vi "Swerve Drive 2 Controller.vi"(8 "error in":errorcluster) -> ()   [LabVIEW 2015]
doc: "This VI executes continuously carrying out the current operation and responding to updates or new operations. It will often contain the timing or control code that is difficult to place directly in TeleOp. This VI generally opens all sensors and motors and isolates the rest of the robot code from knowing how the operations are carried out."
uses:
  <vilib>/Utility/config.llb/NI_LVConfig.lvlib
  <vilib>/Rock Robotics/WPI/CAN/TalonSRX/WPI_CANTalonSRX_APIFeedbackSelect.ctl
  <vilib>/Rock Robotics/WPI/CAN/TalonSRX/WPI_CANTalonSRX_APIControlMode.ctl
  <vilib>/Rock Robotics/WPI/MotorControl/WPI_MotorControlOpenCANTalonSRX.vi
  navX/navX Library v2/navX Library v2.lvlib
  Swerve Drive 2 Operations.ctl
  Swerve Drive 2 Setpoints.ctl
  <vilib>/Utility/config.llb/Read Key (Double).vi
  navX/navX Library v2/IO/Open/Z900_navX_Open_SPI.vi
  <vilib>/Rock Robotics/Network Tables/NT Write Boolean.vi
panel:
  in  "Absolute Encoder TPR":dbl
  out "Joystick":T1
  in  "Speed PID":cluster{"P":dbl, "I":dbl, "D":dbl}={"P"=48.0, "I"=0.0, "D"=638.0}
  in  "Ramp Rate":dbl=50.0
  in  "Steering PID":cluster{"P":dbl, "I":dbl, "D":dbl}={"P"=0.0275, "I"=0.000115, "D"=0.682955}
  out "Current\nCmd":string
  # "Tip: It may be helpful to observe inputs and sensor values.\nYou may also want to display tuning or debugging controls."
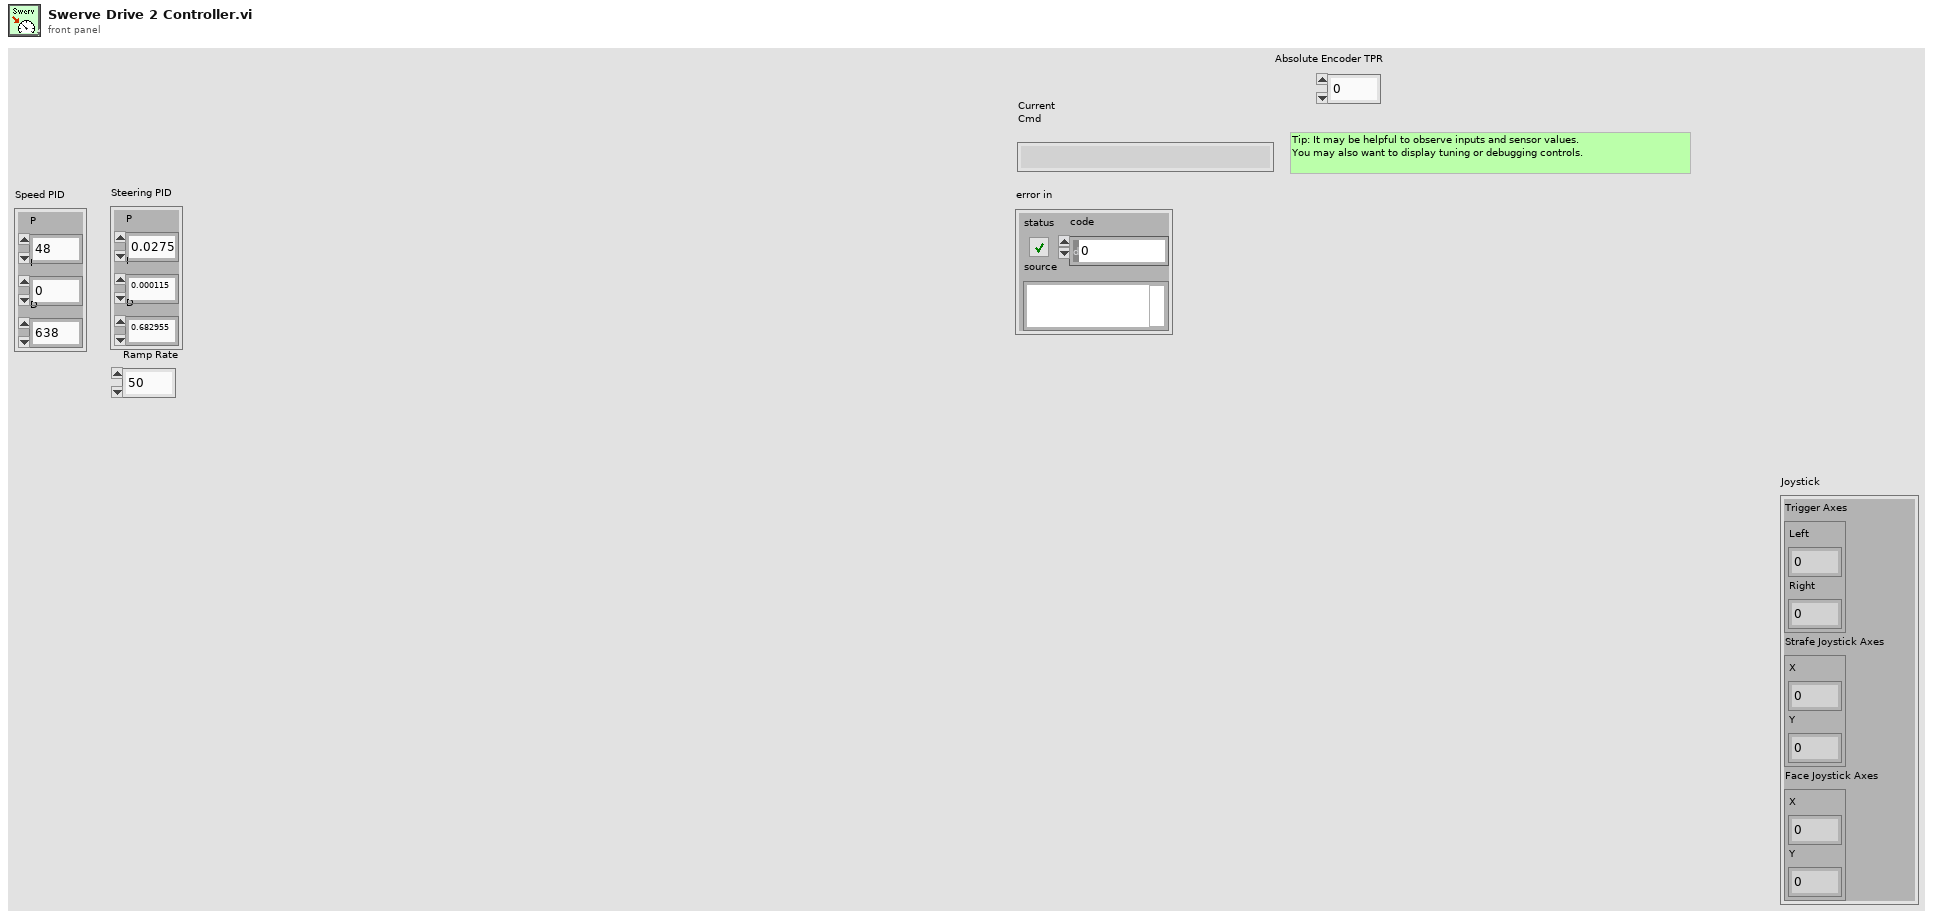
[diagram p1: front panel]
types:
  T1 = cluster{"Trigger Axes":cluster{"Left":dbl, "Right":dbl}, "Strafe Joystick Axes":cluster{"X":dbl, "Y":dbl}, "Face Joystick Axes":cluster{"X":dbl, "Y":dbl}}
  T2 = typedef "Swerve Drive 2 Setpoints.ctl" = cluster{"Operation":T3, "Duration":dbl, "Speed Multiplier":dbl, "Joystick":cluster{"Trigger Axes":cluster{"Left":dbl, "Right":dbl}, "Strafe Joystick Axes":cluster{"X":dbl, "Y":dbl}, "Face Joystick Axes":cluster{"X":dbl, "Y":dbl}}, "Position":cluster{"X":dbl, "Y":dbl, "R":dbl}}
  T3 = typedef "Swerve Drive 2 Operations.ctl" = enum16{"Reserve", "Read Current", "Immeditate", "Drive", "Go to Coordinates"}
  T4 = typedef "NI_LVConfig.lvlib/Config Data RefNum.ctl" = refnum<k1>
  T5 = typedef "WPI_CANTalonSRX_APIFeedbackSelect.ctl" = enum16{"Digital Quadrature Encoder", "Analog Potentiometer", "Analog Encoder", "Count on Quad-A (Rising-Edge)", "Count on Quad-A (Falling-Edge)", "CTR Magnetic Enc (Absolute)", "CTR Magnetic Enc (Relative)", "Pulse Width"}
  T6 = typedef "WPI_CANTalonSRX_APIControlMode.ctl" = enum8{"Percent VBus", "Speed", "Position", "Slave", "Unchanged / Invalid", "Voltage Compensation", "Current"}
  T7 = typedef "WPI_MotorControlDeviceRef.ctl" = cluster{"DeviceStatus":errorcluster, "Type":T8, "PWM":cluster{"PWM Channel":T9, "DeadBand":T10}, "CAN":cluster{"Device Number":u8, "Control Mode":T11, "Semaphore":T12, "Max Vout":dbl, "TalonSRX Control Mode":T6}, "Invert":bool}
  T8 = typedef "WPI_MotorControlType.ctl" = enum16{"PWM", "CAN", "CANTalonSRX"}
  T9 = typedef "FPGA_DIOPWMChannel.ctl" = enum8{"PWM 0", "PWM 1", "PWM 2", "PWM 3", "PWM 4", "PWM 5", "PWM 6", "PWM 7", "PWM 8", "PWM 9", "PWM MXP 0", "PWM MXP 1", "PWM MXP 2", "PWM MXP 3", "PWM MXP 4", "PWM MXP 5", "PWM MXP 6", "PWM MXP 7", "PWM MXP 8", "PWM MXP 9", "Invalid"}
  T10 = typedef "WPI_PWMDeadband.ctl" = cluster{"Name":string, "maxPositivePwm":i32, "minPositivePwm":i32, "centerPwm":i32, "maxNegativePwm":i32, "minNegativePwm":i32, "angularRange":u16}
  T11 = typedef "WPI_CANJaguar_ControlMode.ctl" = enum8{"Percent VBus", "Current", "Speed", "Position", "Voltage"}
  T12 = typedef "Semaphore RefNum" = refnum<k1>
  T13 = cluster{"FL Angle":dbl, "FR Angle":dbl, "RL Angle":dbl, "RR Angle":dbl}
  T14 = cluster{"normalized array[0]":dbl, "normalized array[1]":dbl, "normalized array[2]":dbl, "normalized array[3]":dbl}
  T15 = typedef "Command Status Info.ctl" = cluster{"Name":string, "Status":T16, "notifier out":T17}
  T16 = typedef "Completion Status.ctl" = enum16{"Successful", "Aborted", "Incomplete"}
  T17 = typedef "Completion Notifier.ctl" = refnum<notifier>
  T18 = cluster{"Default Command":T2, "Command Timing":cluster{"Start Time (ms)":u32, "Iterations":i32}, "Command Arguments":cluster{"Command Info":T15, "Description":string, "Default Command":T2, "notifier out":refnum<notifier>, "Subsystem Name":string}}
  T19 = typedef "navX Library v2.lvlib/Z900_navX_DeviceTypeDef.ctl" = cluster{"Interface":cluster{"Protocol":T20, "Update Rate (4Hz-60Hz)":u8, "navX Open TypeDef":variant}, "Notify Packet":refnum<notifier>, "Loop VI Refnum":refnum<vi>, "Ready to Close Occurrence Refnum":refnum<k4>}
  T20 = typedef "navX Library v2.lvlib/Z900_navX_ProtocolTypeDef.ctl" = enum16{"SERIAL", "I2C", "SPI"}
  T21 = cluster{"Yaw":dbl, "Roll":dbl, "Pitch":dbl, "Heading":dbl, "Fused Heading":dbl}
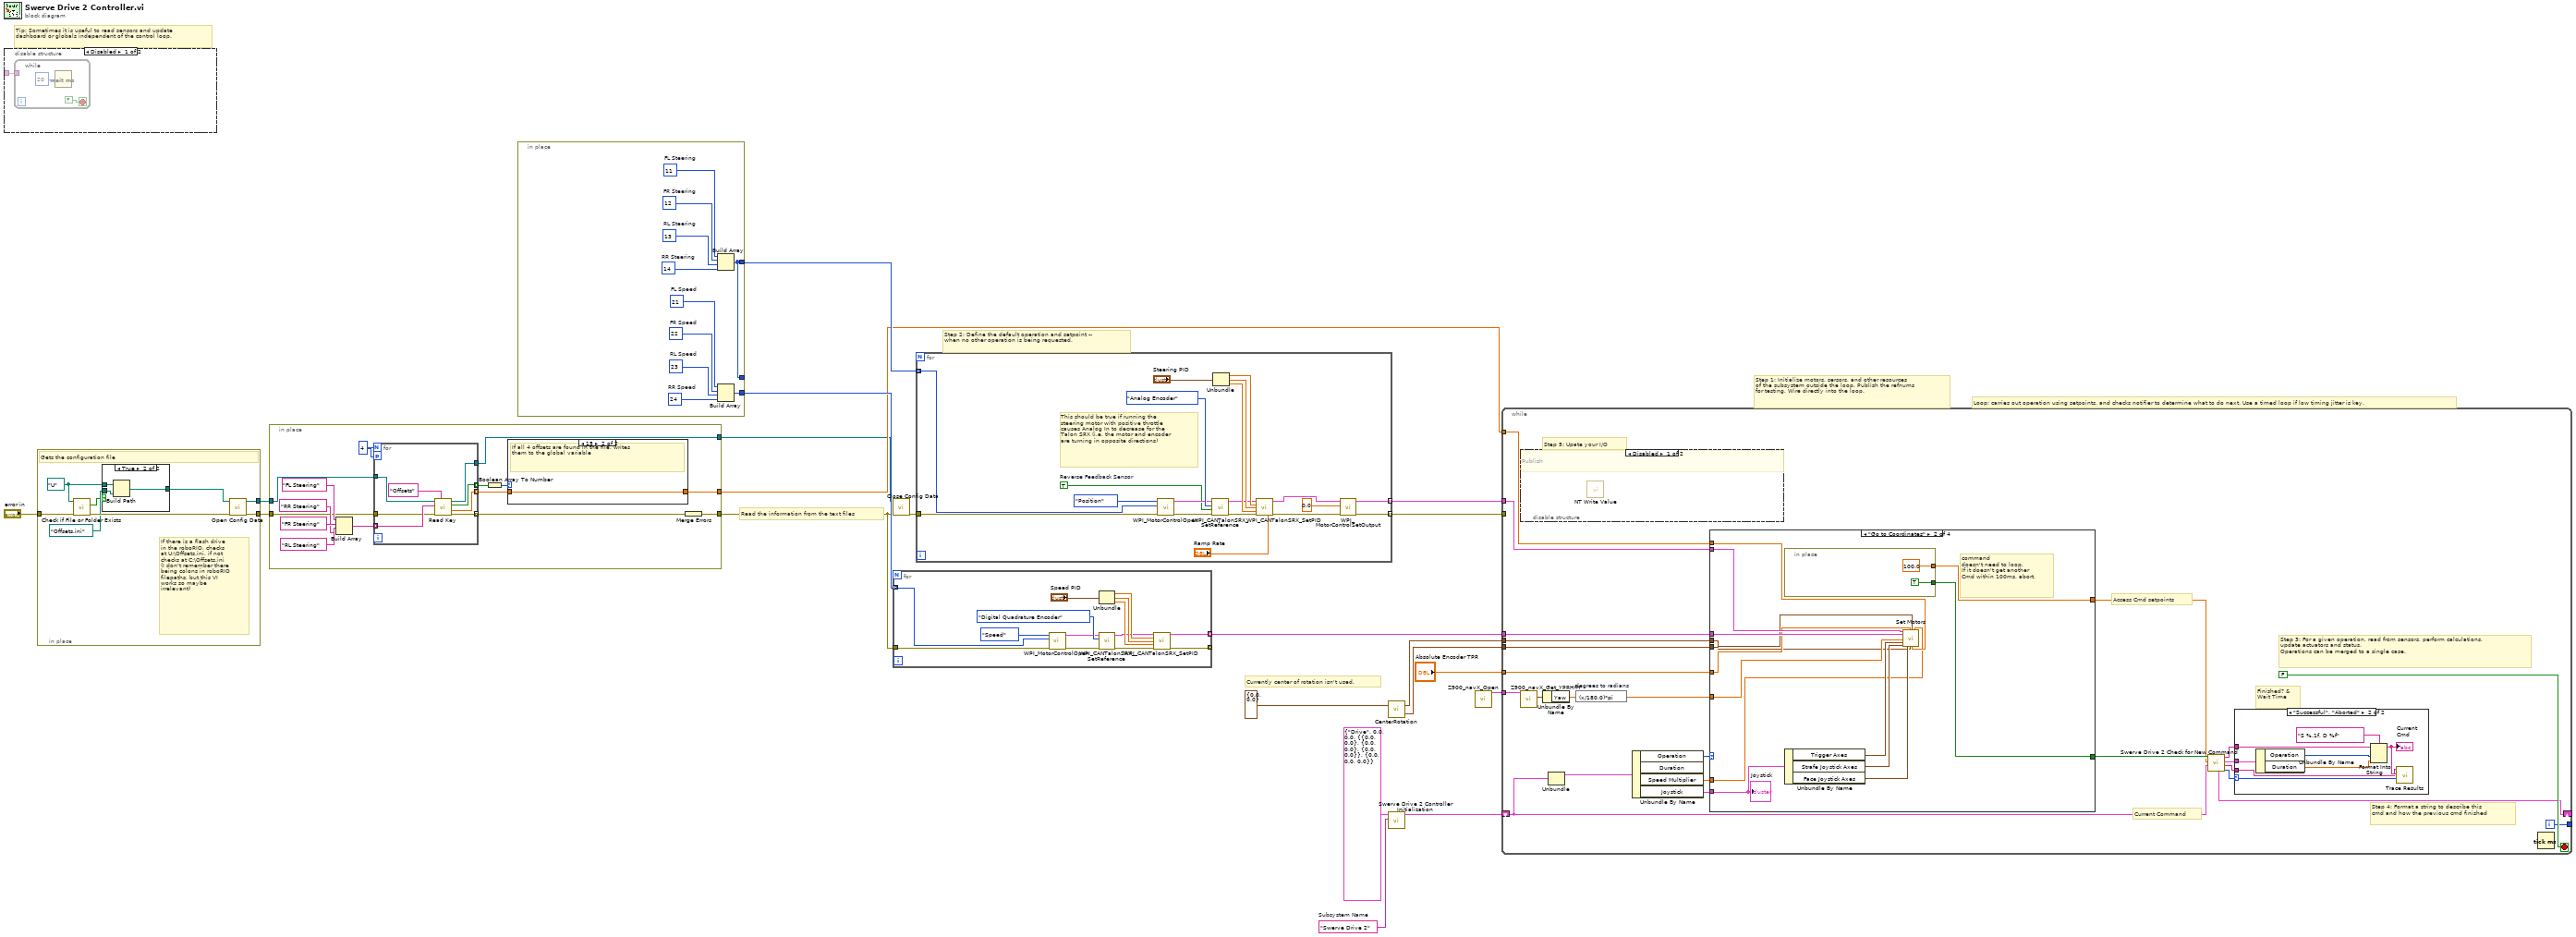
[diagram p0: block diagram]
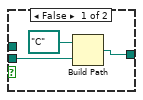
[diagram p2: hidden frame]
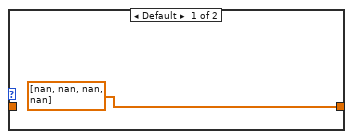
[diagram p3: hidden frame]
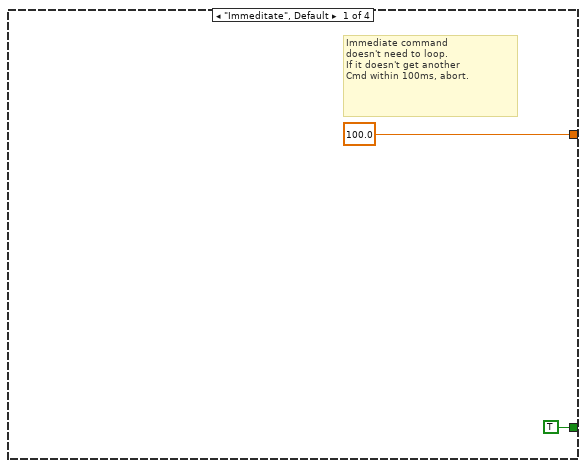
[diagram p5: hidden frame]
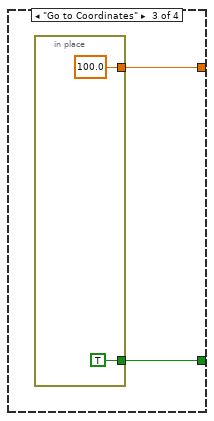
[diagram p6: hidden frame]
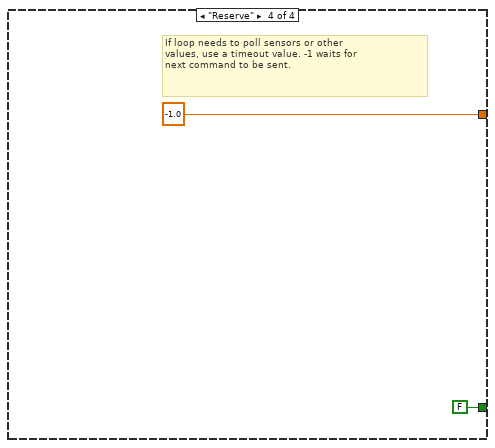
[diagram p7: hidden frame]
diagram:
  w19 = "Swerve Drive 2"  # Subsystem Name
  # "Currently center of rotation isn't used."
  # "Read the information from the text files"
  # "Tip: Sometimes it is useful to read sensors and update\ndashboard or globals independent of the control loop."
  # "Step 2: Define the default operation and setpoint --\nwhen no other operation is being requested."
  # "Step 1: Initialize motors, sersors, and other resources\nof the subsystem outside the loop. Publish the refnums\nfor testing. Wire directly into the loop."
  # "Loop: carries out operation using setpoints, and checks notifier to determine what to do next. Use a timed loop if low timing jitter is key."
  n1 = disable-structure shown="Disabled" {
    disable-tunnel: _ -> [w21 _]
    frame Disabled {
      n2 = while {
        tunnel: w21 -> [_]
        stop <- FALSE stop-if-true
        n3 = Wait (ms)(milliseconds to wait=u32 20) -> ()  [unwired: 1 out]
      }
    }
    frame Enabled {
    }
  }
  n4 = in-place {
    in-place-border: "error in" -> [w31]
    in-place-border: [w29] -> w18
    in-place-border: [w28] -> w17
    w24 = path "U:/" ("base path")
    # "If there is a flash drive\nin the roboRIO, checks\nat U:\\Offsets.ini, if not \nchecks at C:\\Offsets.ini\n(I don't remember there\nbeing colons in roboRIO\nfilepaths, but this VI\nworks so maybe \nirrelevant)"
    # "Gets the configuration file"
    n5 = call <vilib>:"Check if File or Folder Exists.vi"("error in (no error)"=w31, "path"=w24) -> ("error out"=w30:errorcluster, "file or folder exists?"=w25:bool)  [unwired: 7 in, 1 out]
    n6 = case shown="True" w25 {
      tunnel: path "Offsets.ini" ("default name") -> [w34 w35]
      tunnel: [w33 w36] -> w27
      tunnel: w24 -> [_ w37]
      frame False {
        n7 = Build Path(base path=path "C:/", name or relative path=w34) -> (appended path=w33:path)
      }
      frame True {
        n8 = Build Path(base path=w37, name or relative path=w35) -> (appended path=w36:path)
      }
    }
    n9 = call <vilib>:"Open Config Data.vi"("error in (no error)"=w30, "configuration file path"=w27) -> ("error out"=w29:errorcluster, "refnum"=w28:T4)  [unwired: 1 in, 7 out]
  }
  n10 = in-place {
    in-place-border: w18 -> [w42]
    in-place-border: [w40] -> w11
    in-place-border: w17 -> [w41]
    in-place-border: [w39] -> w1
    in-place-border: [w38] -> w9
    w52 = 4
    n11 = Build Array("FL Steering", "FR Steering" ("element"), "RL Steering" ("element"), "RR Steering" ("element")) -> (w47:string[])
    n12 = for {
      N: w52 -> [_]
      workers-P: w52 -> [_]
      tunnel: w47 -> [w62] mode=indexing
      tunnel: w41 -> [w61]
      tunnel: [w60] -> w45 mode=indexing
      tunnel: w42 -> [w59]
      tunnel: [w58] -> w46 mode=indexing
      tunnel: [w57] -> w44 mode=indexing
      tunnel: [w56] -> w39
      n13 = call-poly <vilib>:"Read Key.vi"("section"="Offsets", "error in (no error)"=w59, "key"=w62, "refnum"=w61) -> ("error out"=w58:errorcluster, "value"=w60:dbl, "found?"=w57:bool, "refnum out"=w56:T4)  [unwired: 4 in]
    }
    n14 = Boolean Array To Number(Boolean array=w44) -> (number=w43:u32)
    n15 = case shown="15" w43 {
      tunnel: w45 -> [_ w54]
      tunnel: [dbl[] [nan, nan, nan, nan] w54] -> w38
      frame Default {
      }
      frame 15 {
        # "If all 4 offsets are found in the file, writes\nthem to the global variable"
      }
    }
    n16 = Merge Errors(w46) -> (w40:errorcluster)
  }
  n17 = in-place {
    in-place-border: [w63] -> _
    in-place-border: [w64] -> w12
    in-place-border: [w63] -> w13
    w72 = u8 11  # FL Steering
    w65 = u8 24  # RR Speed
    w66 = u8 23  # RL Speed
    w67 = u8 22  # FR Speed
    w68 = u8 21  # FL Speed
    w69 = u8 14  # RR Steering
    w70 = u8 13  # RL Steering
    w71 = u8 12  # FR Steering
    n18 = Build Array(w72, w71, w70, w69) -> (w63:u8[])
    n19 = Build Array(w68, w67, w66, w65) -> (w64:u8[])
  }
  n20 = call <vilib>:"Close Config Data.vi"("error in (no error)"=w11, "refnum"=w1) -> ("error out"=w15:errorcluster)  [unwired: 8 in, 1 out]
  n21 = for {
    tunnel: w11 -> [w83]
    tunnel: [w75] -> _ mode=indexing
    tunnel: w12 -> [w78] mode=indexing
    tunnel: [w74] -> w7 mode=indexing
    n22 = call-poly <vilib>:"WPI_MotorControlOpen.vi"("error in (no error)"=w83, "Device Number"=w78, "Control Mode"=WPI_CANTalonSRX_APIControlMode."Speed") -> ("error out"=w77:errorcluster, "MotorControlDeviceRef"=w76:T7)  [unwired: 7 in]
    n23 = Unbundle("Speed PID") -> ("P"=w86:dbl, "I"=w85:dbl, "D"=w84:dbl)
    n24 = call <vilib>:"WPI_CANTalonSRX_SetReference.vi"("error in (no error)"=w77, "Feedback Reference"=WPI_CANTalonSRX_APIFeedbackSelect."Digital Quadrature Encoder", "CAN Talon SRX Ref"=w76) -> ("error out"=w81:errorcluster, "CAN Talon SRX Ref Out"=w82:T7)  [unwired: 7 in]
    n25 = call <vilib>:"WPI_CANTalonSRX_SetPID.vi"("CAN Talon SRX Ref"=w82, "P"=w86, "I"=w85, "D"=w84, "error in (no error)"=w81) -> ("CAN Talon SRX Ref Out"=w74:T7, "error out"=w75:errorcluster)  [unwired: 9 in]
  }
  n26 = for {
    tunnel: w15 -> [w102]
    tunnel: w13 -> [w97] mode=indexing
    tunnel: [w90] -> w8 mode=indexing
    tunnel: [w87] -> w14 mode=indexing
    w92 = TRUE  # Reverse Feedback Sensor
    # "This should be true if running the\nsteering motor with positive throttle\ncauses Analog In to decrease for the\nTalon SRX (i.e. the motor and encoder\nare turning in opposite directions)"
    n27 = call-poly <vilib>:"WPI_MotorControlOpen.vi"("error in (no error)"=w102, "Device Number"=w97, "Control Mode"=WPI_CANTalonSRX_APIControlMode."Position") -> ("error out"=w98:errorcluster, "MotorControlDeviceRef"=w94:T7)  [unwired: 7 in]
    n28 = call <vilib>:"WPI_CANTalonSRX_SetReference.vi"("error in (no error)"=w98, "Reverse Feedback Sensor"=w92, "Feedback Reference"=WPI_CANTalonSRX_APIFeedbackSelect."Analog Encoder", "CAN Talon SRX Ref"=w94) -> ("error out"=w101:errorcluster, "CAN Talon SRX Ref Out"=w100:T7)  [unwired: 6 in]
    n29 = Unbundle("Steering PID") -> ("P"=w105:dbl, "I"=w104:dbl, "D"=w103:dbl)
    n30 = call <vilib>:"WPI_CANTalonSRX_SetPID.vi"("CAN Talon SRX Ref"=w100, "P"=w105, "I"=w104, "D"=w103, "error in (no error)"=w101, "Ramp Rate"="Ramp Rate") -> ("CAN Talon SRX Ref Out"=w91:T7, "error out"=w89:errorcluster)  [unwired: 8 in]
    n31 = call <vilib>:"WPI_MotorControlSetOutput.vi"("error in (no error)"=w89, "Output"=0.0, "MotorControlDevRef"=w91) -> ("error out"=w87:errorcluster, "MotorControlDevRef"=w90:T7)  [unwired: 6 in, 1 out]
  }
  n32 = call "CenterRotation.vi"("Center of Rotation Joystick Axes"=cluster{"X":dbl, "Y":dbl} {"X"=0.0, "Y"=0.0}) -> ("Rotation Angle Cluster"=w3:T13, "Rotation Multipliers"=w2:T14)  [unwired: 1 in]
  n33 = call "Swerve Drive 2 Controller Initialization.vi"("Subsystem Name"=w19, "Default Command"=T2 {"Operation"=enum."Drive", "Duration"=0.0, "Speed Multiplier"=0.0, "Joystick"={"Trigger Axes"={"Left"=0.0, "Right"=0.0}, "Strafe Joystick Axes"={"X"=0.0, "Y"=0.0}, "Face Joystick Axes"={"X"=0.0, "Y"=0.0}}, "Position"={"X"=0.0, "Y"=0.0, "R"=0.0}}) -> ("Command Info"=w20:T18)  [unwired: 9 in]
  n34 = call-poly "Z900_navX_Open.vi"() -> ("navX Device"=w6:T19)  [unwired: 10 in, 1 out]
  n35 = while {
    shift-right: [w125] -> _
    shift-left: w20 -> [w126]
    tunnel: [w128] -> _
    tunnel: w14 -> [_]
    tunnel: "Absolute Encoder TPR" -> [w119]
    tunnel: w9 -> [w118]
    tunnel: w8 -> [w117]
    tunnel: w7 -> [w116]
    tunnel: w6 -> [w113]
    tunnel: w3 -> [w109]
    tunnel: w2 -> [w108]
    i -> [w128]
    stop <- FALSE stop-if-true
    # "Step 5: Upate your I/O"
    # "Step 4: Format a string to describe this\ncmd and how the previous cmd finished"
    # "Current Command"
    # "Access Cmd setpoints"
    # "Finished? &\nWait Time"
    # "Step 3: For a given operation, read from sensors, perform calculations,\nupdate actuators and status.\nOperations can be merged to a single case."
    n36 = disable-structure shown="Disabled" {
      frame Disabled {
        # "Publish"
        n37 = call-poly <vilib>:"NT Write Value.vi"() -> ()  [unwired: 11 in, 1 out]
      }
      frame Enabled {
      }
    }
    n38 = call "Z900_navX_Get_YPRHfH.vi"("navX Device"=w113) -> ("YRPHfH"=w115:T21)  [unwired: 7 in, 3 out]
    n39 = Unbundle By Name(w115) -> ("Yaw"=w114:dbl)
    n40 = Unbundle(w126) -> ("Default Command"=w127:T2)  [unwired: 2 out]
    n41 = expression code="(x/180.0)*pi" "degrees to radians"(w114) -> (w112:dbl)
    n42 = Unbundle By Name(w127) -> ("Operation"=w120:T3, "Speed Multiplier"=w110:dbl, "Joystick"=w111:T1)  [unwired: 1 out]
    n43 = case shown="\"Go to Coordinates\"" w120 {
      tunnel: [100.0 w144 w149 -1.0] -> w106
      tunnel: [TRUE ("ignore previous (F)") w145 w148 FALSE ("ignore previous (F)")] -> w107
      tunnel: w116 -> [_ w140 _ _]
      tunnel: w117 -> [_ w141 _ _]
      tunnel: w111 -> [_ w143 _ _]
      tunnel: w109 -> [_ w137 _ _]
      tunnel: w112 -> [_ w136 _ _]
      tunnel: w118 -> [_ w135 _ _]
      tunnel: w119 -> [_ w134 _ _]
      tunnel: w110 -> [_ w133 _ _]
      tunnel: w108 -> [_ w132 _ _]
      frame "Immeditate", Default {
        # "Immediate command\ndoesn't need to loop.\nIf it doesn't get another\nCmd within 100ms, abort."
      }
      frame "Go to Coordinates" {
        # "command\ndoesn't need to loop.\nIf it doesn't get another\nCmd within 100ms, abort."
        n44 = in-place {
          in-place-border: [TRUE ("ignore previous (F)")] -> w145
          in-place-border: [100.0] -> w144
        }
        n45 = Unbundle By Name(w143) -> ("Trigger Axes"=w142:cluster{"Left":dbl, "Right":dbl}, "Strafe Joystick Axes"=w139:cluster{"X":dbl, "Y":dbl}, "Face Joystick Axes"=w138:cluster{"X":dbl, "Y":dbl})
        n46 = call "Set Motors.vi"("Position Motors"=w141, "Speed Motors"=w140, "Angle (radians; 0 = right)"=w136, "Trigger Axes"=w142, "Strafe Joystick Axes"=w139, "Face Joystick Axes"=w138, "Absolute Encoder TPR"=w134, "Rotation Multipliers"=w132, "Rotation Angle Cluster"=w137, "Drive Train Absolute Offsets (ticks)"=w135, "Speed Multipliers"=w133) -> ()  [unwired: 8 in, 1 out]
        "Joystick" <- w143
      }
      frame "Go to Coordinates" {
        n47 = in-place {
          in-place-border: [TRUE ("ignore previous (F)")] -> w148
          in-place-border: [100.0] -> w149
        }
      }
      frame "Reserve" {
        # "If loop needs to poll sensors or other\nvalues, use a timeout value. -1 waits for\nnext command to be sent."
      }
    }
    n48 = call "Swerve Drive 2 Check for New Command.vi"("Current Command"=w126, "Wait time (ms)"=w106, "Finished?"=w107) -> ("Completion"=w121:T16, "Subsystem Name"=w122:string, "Current Command"=w123:T2, "Initial Trace String"=w124:string, "NextCommand"=w125:T18)  [unwired: 4 in]
    n49 = case shown="\"Successful\", \"Aborted\"" w121 {
      selector: w121 -> [_ w161]
      tunnel: w124 -> [_ w158]
      tunnel: w123 -> [_ w159]
      tunnel: w122 -> [_ w155]
      frame "Incomplete", Default {
        # "Continuing current command"
      }
      frame "Successful", "Aborted" {
        # "Report and setup for next command"
        n50 = Unbundle By Name(w159) -> ("Operation"=w154:T3, "Duration"=w156:dbl)
        n51 = Format Into String(format string="S %.1f, D %f", initial string=w158, w154, w156) -> (resulting string=w157:string)  [unwired: 1 in, 1 out]
        "Current\nCmd" <- w157
        n52 = call "Trace Results.vi"("Status of previous command"=w161, "Description"=w157, "Subsystem"=w155) -> ()  [unwired: 9 in]
      }
    }
    n53 = Tick Count (ms)() -> ()  [unwired: 1 out]
  }
